vi "pcap close.vi"(8 "error in":errorcluster, 11 "pcap_t in":u64) -> (0 "error out":errorcluster)   [LabVIEW 2020, in "libpcaplv.lvlib"]
uses:
  libpcaplv.lvlib
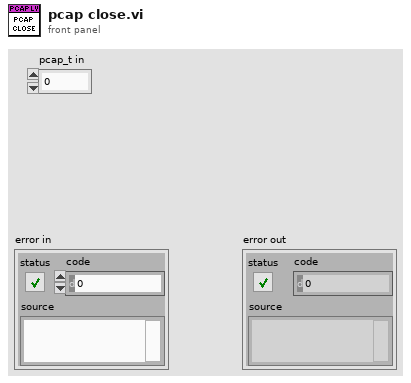
[diagram p1: front panel]
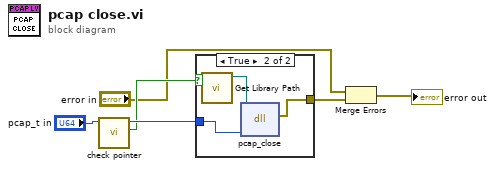
[diagram p0: block diagram]
diagram:
  n1 = call "check pointer.vi"("pointer in"="pcap_t in") -> ("ok"=w5:bool, "pointer out"=w6:u64)  [unwired: 9 in]
  n2 = case shown="True" w5 {
    tunnel: [_ w8] -> w3
    tunnel: w6 -> [_ w9]
    frame False {
    }
    frame True {
      n3 = call "Get Library Path.vi"() -> ("library path"=w7:path)  [unwired: 11 in]
      n4 = dll-call lib="libpcap.*" fn="pcap_close"(path in=w7, "pcap_t"=w9) -> (error out=w8:errorcluster)  [unwired: 4 in, 1 out]
    }
  }
  n5 = Merge Errors("error in", w3) -> (→"error out":errorcluster)
